vi "EnableDisable - Right Click.vi"(8 "error in (no error)":errorcluster, 11 "Node Ptr":u64 format="%.0x") -> (0 "error out":errorcluster)   [LabVIEW 2015, in "Engine Simulation Toolkit System Explorer.lvlib"]
uses:
  Engine Simulation Toolkit System Explorer.lvlib
  Shared/Constants and GUIDs.vi
  <vilib>/NI Veristand/Custom Device API/Custom Device API.lvlib
  Shared/Engine Simulation Toolkit Shared.lvlib
panel:
  in  "Tag":string
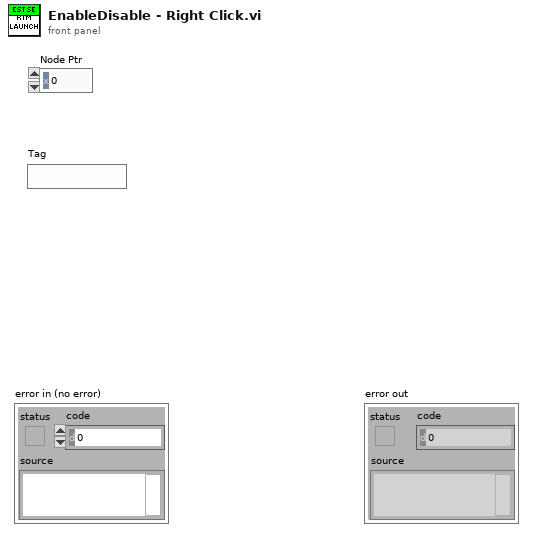
[diagram p1: front panel]
types:
  T1 = typedef "Custom Device API.lvlib/Custom Device Item Ref.ctl" = u64
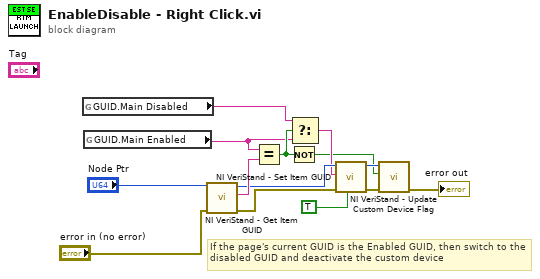
[diagram p0: block diagram]
diagram:
  # "If the page's current GUID is the Enabled GUID, then switch to the disabled GUID and deactivate the custom device"
  n1 = global read "Constants and GUIDs.vi" "GUID.Main Disabled"() -> (w2:string)
  n2 = global read "Constants and GUIDs.vi" "GUID.Main Enabled"() -> (w1:string)
  n3 = call <vilib>:"NI VeriStand - Get Item GUID.vi"("error in (no error)"="error in (no error)", "Item Ref in"="Node Ptr") -> ("error out"=w12:errorcluster, "GUID"=w14:string, "Item Ref out"=w11:T1)  [unwired: 7 in]
  n4 = Equal?(x=w1, y=w14) -> (x = y?=w7:bool)
  n5 = Not(x=w7) -> (.not. x?=w6:bool)
  n6 = Select(t=w2, s=w7, f=w1) -> (s? t:f=w10:string)
  n7 = call <vilib>:"NI VeriStand - Set Item GUID.vi"("Refresh System Explorer Tree? (F)"=TRUE, "error in (no error)"=w12, "GUID"=w10, "Item Ref in"=w11) -> ("error out"=w9:errorcluster, "Item Ref out"=w8:T1)  [unwired: 6 in]
  n8 = call <vilib>:"NI VeriStand - Update Custom Device Flag.vi"("error in (no error)"=w9, "Is Custom Device Active?"=w6, "Device Ref in"=w8) -> ("error out"=→"error out":errorcluster)  [unwired: 7 in, 1 out]
